vi "CalculateCCDReadoutTime.vi"(1 "Color":string, 2 "Readout Speed":dbl, 3 "CCD ROI":cluster{i32, i32, i32, i32, i32, i32}) -> (0 "Readout Time":dbl)   [LabVIEW 2015]
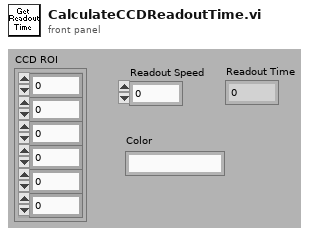
[diagram p1: front panel]
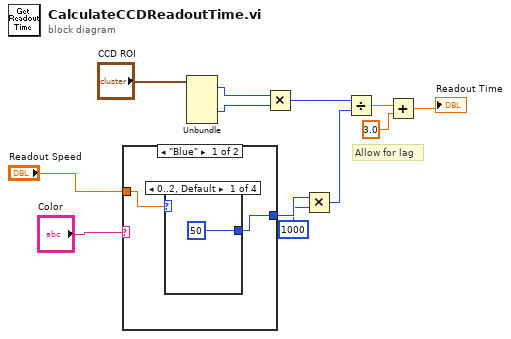
[diagram p0: block diagram]
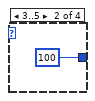
[diagram p2: hidden frame]
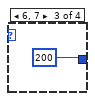
[diagram p3: hidden frame]
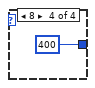
[diagram p4: hidden frame]
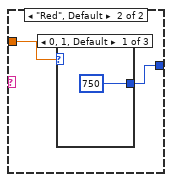
[diagram p5: hidden frame]
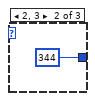
[diagram p6: hidden frame]
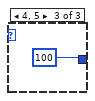
[diagram p7: hidden frame]
diagram:
  # "Allow for lag"
  n1 = case shown="\"Blue\"" "Color" {
    tunnel: "Readout Speed" -> [w13 w20]
    tunnel: [w14 w19] -> w10
    frame "Blue" {
      n2 = case shown="0..2, Default" w13 {
        tunnel: [50 100 200 400] -> w14
        frame 0..2, Default {
        }
        frame 3..5 {
        }
        frame 6, 7 {
        }
        frame 8 {
        }
      }
    }
    frame "Red", Default {
      n3 = case shown="0, 1, Default" w20 {
        tunnel: [750 344 100] -> w19
        frame 0, 1, Default {
        }
        frame 2, 3 {
        }
        frame 4, 5 {
        }
      }
    }
  }
  n4 = Unbundle("CCD ROI") -> (w6:i32, w5:i32)  [unwired: 4 out]
  n5 = Multiply(x=w6, y=w5) -> (x*y=w8:i32)
  n6 = Multiply(x=w10, y=1000) -> (x*y=w7:i32)
  n7 = Divide(x=w8, y=w7) -> (x/y=w4:dbl)
  n8 = Add(x=w4, y=3.0) -> (x+y=→"Readout Time":dbl)
